vi "Meas Get Record Section.vi"(5 "record index ref":refnum<vi>, 7 "grp index ref":refnum<vi>, 8 "error in":errorcluster, 9 "sub-rec index ref":refnum<vi>, 10 "source mode":T1, 11 "record info":T2={"header path"=path "", "group id"=0, "average id"=0, "Time Stamp"=timestamp(0 s since 1904-01-01), "max samples"=0, "first sample"=0, "first smpl [%]"=-1.0, "kill viewer"=FALSE}) -> (0 "error out":errorcluster, 1 "record path":path, 2 "time [s]":dbl[](array[numeric]), 3 "waveforms [V]":sgl[][](array[numeric]), 4 "labels":string[](array[string]))   [LabVIEW 2020]
doc: "Reads desired section of the record defined in 'record info'. It will read the header file, it will parse it in order to find particular record in it, then it fetches desired portion of the sample data from binary sample file. Then it scales the data using scale factors from the header file."
uses:
  GUI/GUI Waveform Info.ctl
  Meas Sample Reader Source Mode.ctl
  8804b04d-be98-4d58-8b56-90ec7a7b7f07.vi
  octave/infolib/GetI64.vi
  octave/infolib/Get 1D String.vi
  octave/infolib/GetString.vi
  octave/infolib/Get 1D I64.vi
  <vilib>/Comparison/Equal/Equal Functor/Equal Functor.lvclass
  octave/infolib/infolib.lvlib
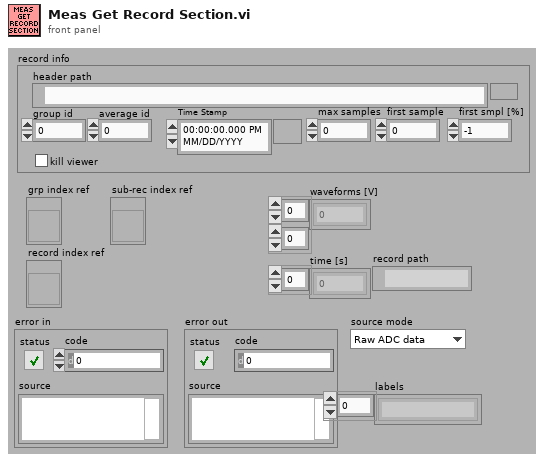
[diagram p1: front panel]
types:
  T1 = typedef "Meas Sample Reader Source Mode.ctl" = enum16{"Raw ADC data", "Transducers"}
  T2 = typedef "GUI Waveform Info.ctl" = cluster{"header path":path, "group id":i32, "average id":i32, "Time Stamp":timestamp, "max samples":i64, "first sample":i64, "first smpl [%]":dbl, "kill viewer":bool}
  T3 = typedef "Corr Transducer INFO Record.ctl" = cluster{"name":string, "serial":string, "channel name":string, "items":T4[], "type":string}
  T4 = typedef "Corr Transducer INFO Item.ctl" = cluster{"name":string, "is numeric":bool, "value":dbl, "uncertainty":dbl, "string value":string, "template":T5, "info":string}
  T5 = typedef "Corr CSV Template.ctl" = cluster{"quantities":string[], "y-axis":string, "x-axis":string}
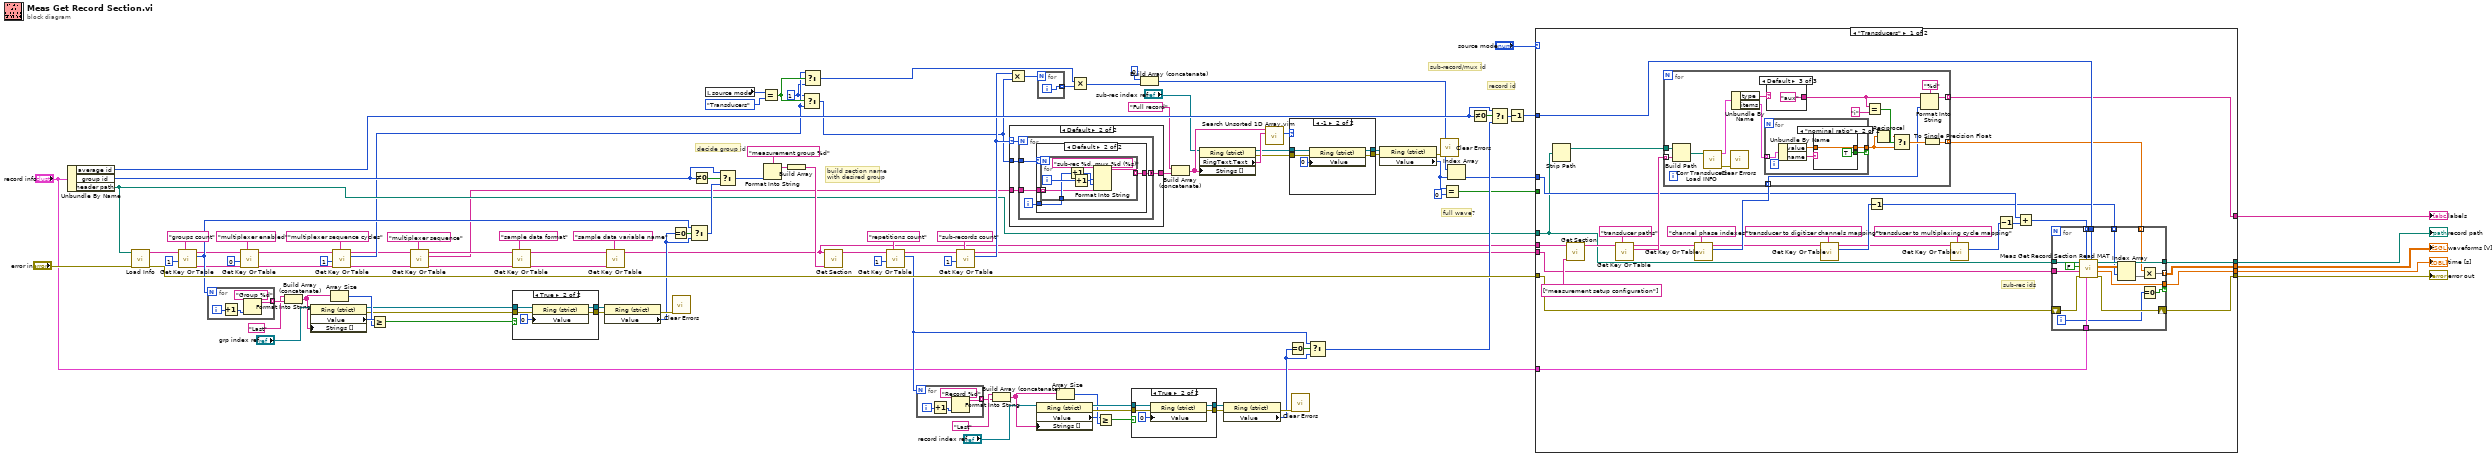
[diagram p0: block diagram]
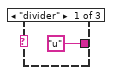
[diagram p3: hidden frame]
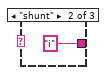
[diagram p4: hidden frame]
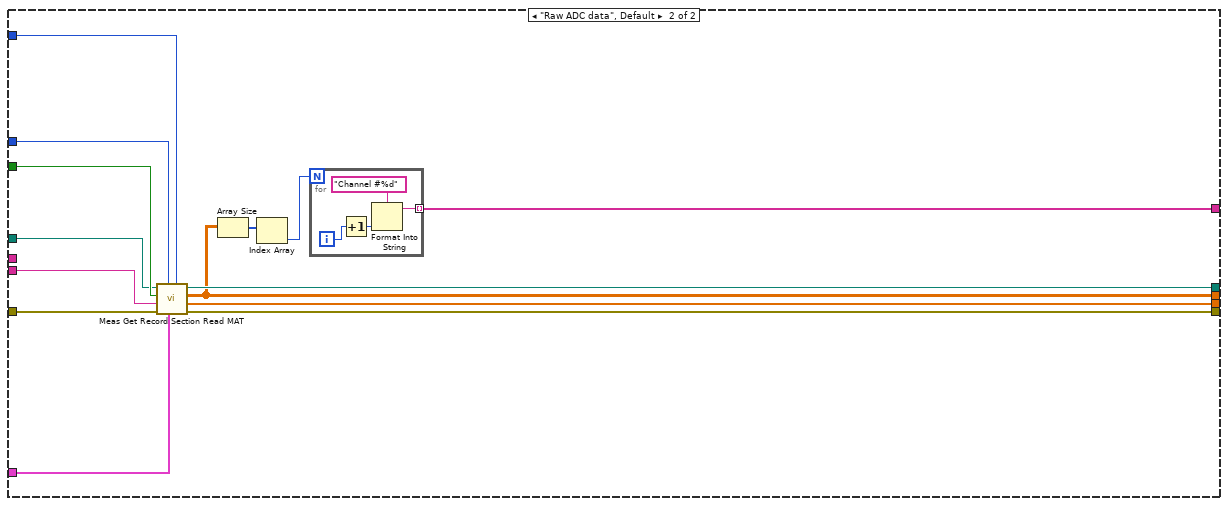
[diagram p5: hidden frame]
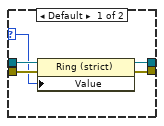
[diagram p6: hidden frame]
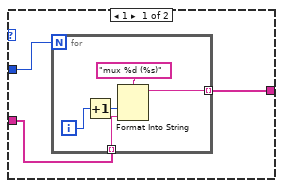
[diagram p7: hidden frame]
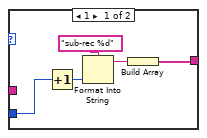
[diagram p8: hidden frame]
diagram:
  w10 = i64 1 ("t")
  # "full wave?"
  # "sub-record/mux id"
  # "record id"
  # "decide group id"
  # "build section name\nwith desired group"
  n1 = Unbundle By Name("record info") -> ("average id"=w97:i32, "group id"=w102:i32, "header path"=w18:path)
  n2 = call "Load Info.vi"("error in"="error in", "filename"=w18) -> ("error out"=w90:errorcluster, "info data"=w106:string)  [unwired: 8 in]
  n3 = call-poly "Get Key Or Table.vi"("key description"="groups count", "numeric"=i64 1, "info data"=w106) -> ("sections out"=w52:string[], "value"=w59:i64, "info data out"=w51:string)  [unwired: 5 in, 1 out]
  n4 = for {
    N: w59 -> [_]
    tunnel: [w111] -> w85 mode=indexing
    i -> [w113]
    n5 = Increment(x=w113) -> (x+1=w110:i32)
    n6 = Format Into String(format string="Group %d", w110) -> (resulting string=w111:string)  [unwired: 2 in, 1 out]
  }
  n7 = call-poly "Get Key Or Table.vi"("key description"="multiplexer enabled", "sections"=w52, "numeric"=i64 0, "info data"=w51) -> ("sections out"=w47:string[], "info data out"=w48:string)  [unwired: 4 in, 2 out]
  n8 = Build Array (concatenate)("Last", w85) -> (w82:string[])
  n9 = property class="Ring (strict)"(reference="grp index ref", "Strings []"=w82) -> (reference out=w80:refnum<vi>, error out=w76:errorcluster, "Value"=w83:u16)  [unwired: 1 in]
  n10 = Array Size(array=w82) -> (size(s)=w81:i32)
  n11 = call-poly "Get Key Or Table.vi"("key description"="multiplexer sequence cycles", "sections"=w47, "numeric"=i64 1, "info data"=w48) -> ("sections out"=w6:string[], "value"=w11:i64, "info data out"=w5:string)  [unwired: 4 in, 1 out]
  n12 = Greater Or Equal?(x=w83, y=w81) -> (x >= y?=w79:bool)
  n13 = call-poly "Get Key Or Table.vi"("key description"="multiplexer sequence", "sections"=w6, "info data"=w5) -> ("sections out"=w3:string[], "value"=w1:string[], "info data out"=w2:string)  [unwired: 5 in, 1 out]
  n14 = call-poly "Get Key Or Table.vi"("key description"="sample data format", "sections"=w3, "info data"=w2) -> ("sections out"=w93:string[], "info data out"=w94:string)  [unwired: 5 in, 2 out]
  n15 = case shown="True" w79 {
    tunnel: w80 -> [w115 w120]
    tunnel: [w115 w118] -> w78
    tunnel: [w114 w117] -> w77
    tunnel: w76 -> [w114 w116]
    frame False {
    }
    frame True {
      n16 = property class="Ring (strict)"(reference=w120, error in=w116, "Value"=u16 0) -> (reference out=w118:refnum<vi>, error out=w117:errorcluster)
    }
  }
  n17 = property class="Ring (strict)"(reference=w78, error in=w77) -> (error out=w75:errorcluster, "Value"=w61:u16)  [unwired: 1 out]
  n18 = call-poly "Get Key Or Table.vi"("key description"="sample data variable name", "sections"=w93, "info data"=w94) -> ("info data out"=w7:string)  [unwired: 5 in, 3 out]
  n19 = Equal To 0?(x=w61) -> (x = 0?=w62:bool)
  n20 = call <vilib>:"Clear Errors.vi"("error in (no error)"=w75) -> ()  [unwired: 5 in, 2 out]
  n21 = Select(t=w59, s=w62, f=w61) -> (s? t:f=w60:i64)
  n22 = Not Equal To 0?(x=w102) -> (x != 0?=w103:bool)
  n23 = local read "source mode"() -> (w14:T1)
  n24 = Select(t=w102, s=w103, f=w60) -> (s? t:f=w101:i64)
  n25 = Equal?(x=w14, y=Meas_Sample_Reader_Source_Mode."Transducers") -> (x = y?=w12:bool)
  n26 = Format Into String(format string="measurement group %d", w101) -> (resulting string=w105:string)  [unwired: 2 in, 1 out]
  n27 = Build Array(w105) -> (w23:string[])
  n28 = Select(t=w10, s=w12, f=w11) -> (s? t:f=w15:i64)
  n29 = Select(t=w11, s=w12, f=w10) -> (s? t:f=w8:i64)
  n30 = call "Get Section.vi"("sections"=w23, "info data"=w7) -> ("section part"=w22:string)  [unwired: 7 in, 2 out]
  n31 = call-poly "Get Key Or Table.vi"("key description"="repetitions count", "numeric"=i64 1, "info data"=w22) -> ("value"=w55:i64, "info data out"=w44:string)  [unwired: 5 in, 2 out]
  n32 = for {
    N: w55 -> [_]
    tunnel: [w122] -> w64 mode=indexing
    i -> [w124]
    n33 = Increment(x=w124) -> (x+1=w121:i32)
    n34 = Format Into String(format string="Record %d", w121) -> (resulting string=w122:string)  [unwired: 2 in, 1 out]
  }
  n35 = call-poly "Get Key Or Table.vi"("key description"="sub-records count", "numeric"=i64 1, "info data"=w44) -> ("value"=w31:i64, "info data out"=w21:string)  [unwired: 5 in, 2 out]
  n36 = Build Array (concatenate)("Last", w64) -> (w67:string[])
  n37 = Multiply(x=w31, y=w15) -> (x*y=w30:i64)
  n38 = case shown="Default" w31 {
    selector: w31 -> [_ w135]
    tunnel: w15 -> [w125 w136]
    tunnel: [w127 w134] -> w43
    tunnel: w1 -> [w126 w133]
    frame 1 {
      n39 = for {
        N: w125 -> [_]
        tunnel: [w130] -> w127 mode=indexing
        tunnel: w126 -> [w128] mode=indexing
        i -> [w129]
        n40 = Increment(x=w129) -> (x+1=w132:i32)
        n41 = Format Into String(format string="mux %d (%s)", w132, w128) -> (resulting string=w130:string)  [unwired: 2 in, 1 out]
      }
    }
    frame Default {
      n42 = for {
        N: w135 -> [_]
        tunnel: w136 -> [w140]
        tunnel: [w138] -> w134 mode=concatenating
        tunnel: w133 -> [w137]
        i -> [w139]
        n43 = case shown="Default" w140 {
          selector: w140 -> [_ w149]
          tunnel: w139 -> [w141 w147]
          tunnel: [w142 w148] -> w138
          tunnel: w137 -> [_ w146]
          frame 1 {
            n44 = Increment(x=w141) -> (x+1=w144:i32)
            n45 = Format Into String(format string="sub-rec %d", w144) -> (resulting string=w143:string)  [unwired: 2 in, 1 out]
            n46 = Build Array(w143) -> (w142:string[])
          }
          frame Default {
            n47 = for {
              N: w149 -> [_]
              tunnel: [w154] -> w148 mode=indexing
              tunnel: w147 -> [w151]
              tunnel: w146 -> [w150] mode=indexing
              i -> [w156]
              n48 = Increment(x=w151) -> (x+1=w152:i32)
              n49 = Increment(x=w156) -> (x+1=w153:i32)
              n50 = Format Into String(format string="sub-rec %d, mux %d (%s)", w152, w153, w150) -> (resulting string=w154:string)  [unwired: 2 in, 1 out]
            }
          }
        }
      }
    }
  }
  n51 = property class="Ring (strict)"(reference="record index ref", "Strings []"=w67) -> (reference out=w69:refnum<vi>, error out=w73:errorcluster, "Value"=w66:u16)  [unwired: 1 in]
  n52 = for {
    N: w30 -> [_]
    tunnel: [w157] -> w29 mode=indexing
    i -> [w157]
  }
  n53 = Array Size(array=w67) -> (size(s)=w68:i32)
  n54 = Multiply(x=w8, y=w29) -> (x*y=w9:i64[])
  n55 = Greater Or Equal?(x=w66, y=w68) -> (x >= y?=w70:bool)
  n56 = case shown="True" w70 {
    tunnel: w69 -> [w159 w164]
    tunnel: [w159 w162] -> w71
    tunnel: [w158 w161] -> w72
    tunnel: w73 -> [w158 w160]
    frame False {
    }
    frame True {
      n57 = property class="Ring (strict)"(reference=w164, error in=w160, "Value"=u16 0) -> (reference out=w162:refnum<vi>, error out=w161:errorcluster)
    }
  }
  n58 = Build Array (concatenate)(0, w9) -> (w28:i64[])
  n59 = Build Array (concatenate)("Full record", w43) -> (w41:string[])
  n60 = property class="Ring (strict)"(reference="sub-rec index ref", "Strings []"=w41) -> (reference out=w36:refnum<vi>, error out=w37:errorcluster, "RingText.Text"=w40:string)  [unwired: 1 in]
  n61 = property class="Ring (strict)"(reference=w71, error in=w72) -> (error out=w74:errorcluster, "Value"=w56:u16)  [unwired: 1 out]
  n62 = call "Search Unsorted 1D Array.vim"("element"=w40, "unsorted 1D array"=w41) -> ("index of element"=w39:i32)  [unwired: 9 in]
  n63 = Equal To 0?(x=w56) -> (x = 0?=w57:bool)
  n64 = case shown="-1" w39 {
    selector: w39 -> [w167 _]
    tunnel: w37 -> [w169 w174]
    tunnel: w36 -> [w168 w173]
    tunnel: [w166 w170] -> w35
    tunnel: [w165 w171] -> w34
    frame Default {
      n65 = property class="Ring (strict)"(reference=w168, error in=w169, "Value"=w167) -> (reference out=w165:refnum<vi>, error out=w166:errorcluster)
    }
    frame -1 {
      n66 = property class="Ring (strict)"(reference=w173, error in=w174, "Value"=u16 0) -> (reference out=w171:refnum<vi>, error out=w170:errorcluster)
    }
  }
  n67 = call <vilib>:"Clear Errors.vi"("error in (no error)"=w74) -> ()  [unwired: 5 in, 2 out]
  n68 = Select(t=w55, s=w57, f=w56) -> (s? t:f=w58:i64)
  n69 = property class="Ring (strict)"(reference=w34, error in=w35) -> (error out=w33:errorcluster, "Value"=w27:u16)  [unwired: 1 out]
  n70 = call <vilib>:"Clear Errors.vi"("error in (no error)"=w33) -> ()  [unwired: 5 in, 2 out]
  n71 = Equal?(x=w27, y=u16 0) -> (x = y?=w19:bool)
  n72 = Index Array(array=w28, index=w27) -> (element=w24:i64)
  n73 = Not Equal To 0?(x=w97) -> (x != 0?=w98:bool)
  n74 = Select(t=w97, s=w98, f=w58) -> (s? t:f=w91:i64)
  n75 = Decrement(x=w91) -> (x-1=w25:i64)
  n76 = case shown="\"Transducers\"" "source mode" {
    tunnel: [w181 w262] -> w92
    tunnel: w90 -> [w187 w261]
    tunnel: [w177 w260] -> w89
    tunnel: [w178 w252] -> w88
    tunnel: [w175 w259] -> w87
    tunnel: w25 -> [w185 w258]
    tunnel: w24 -> [w189 w257]
    tunnel: w21 -> [w183 w256]
    tunnel: "record info" -> [w182 w255]
    tunnel: w19 -> [_ w254]
    tunnel: w18 -> [w184 w253]
    tunnel: [w176 w249] -> w16
    tunnel: w7 -> [w204 _]
    frame "Transducers" {
      # "sub-rec ids"
      n77 = Strip Path(path=w184) -> (stripped path=w201:path)  [unwired: 1 out]
      n78 = call "Get Section.vi"("sections"=string[] ["measurement setup configuration"], "info data"=w204) -> ("section part"=w197:string)  [unwired: 7 in, 2 out]
      n79 = call-poly "Get Key Or Table.vi"("key description"="transducer paths", "info data"=w197) -> ("value"=w200:string[], "info data out"=w198:string)  [unwired: 6 in, 2 out]
      n80 = call-poly "Get Key Or Table.vi"("key description"="channel phase indexes", "info data"=w198) -> ("value"=w196:i64[], "info data out"=w194:string)  [unwired: 6 in, 2 out]
      n81 = for {
        tunnel: w201 -> [w238]
        tunnel: w200 -> [w237] mode=indexing
        tunnel: [w222] -> w179 mode=indexing
        tunnel: w196 -> [w224] mode=indexing
        tunnel: [w223] -> w176 mode=indexing
        n82 = Build Path(base path=w238, name or relative path=w237) -> (appended path=w236:path)
        n83 = call "Corr Transducers Load INFO.vi"("Path"=w236) -> ("error out"=w235:errorcluster, "transducer info"=w234:T3)  [unwired: 9 in]
        n84 = call <vilib>:"Clear Errors.vi"("error in (no error)"=w235) -> ()  [unwired: 5 in, 2 out]
        n85 = Unbundle By Name(w234) -> ("type"=w233:string, "items"=w232:T4[])
        n86 = for {
          tunnel: w232 -> [w243] mode=indexing
          tunnel: [w240] -> w228 if=w239
          n87 = Unbundle By Name(w243) -> ("value"=w241:dbl, "name"=w242:string)
          n88 = case shown="\"nominal ratio\"" w242 {
            tunnel: w241 -> [_ w245]
            tunnel: [_ w245] -> w240
            tunnel: [_ TRUE] -> w239
            frame Default {
            }
            frame "nominal ratio" {
            }
          }
        }
        n89 = case shown="Default" w233 {
          tunnel: ["u" "i" "aux"] -> w226
          frame "divider" {
          }
          frame "shunt" {
          }
          frame Default {
          }
        }
        n90 = Equal?(x=w226, y="i") -> (x = y?=w230:bool)
        n91 = Reciprocal(x=w228) -> (1/x=w229:dbl)
        n92 = Select(t=w229, s=w230, f=w228) -> (s? t:f=w227:dbl)
        n93 = Format Into String(format string="%d", initial string=w226, w224) -> (resulting string=w223:string)  [unwired: 1 in, 1 out]
        n94 = To Single Precision Float(number=w227) -> (single precision float=w222:sgl)
      }
      n95 = call-poly "Get Key Or Table.vi"("key description"="transducer to digitizer channels mapping", "info data"=w194) -> ("value"=w193:i64[], "info data out"=w190:string)  [unwired: 6 in, 2 out]
      n96 = Decrement(x=w193) -> (x-1=w180:i64[])
      n97 = call-poly "Get Key Or Table.vi"("key description"="transducer to multiplexing cycle mapping", "info data"=w190) -> ("value"=w192:i64[])  [unwired: 6 in, 3 out]
      n98 = Decrement(x=w192) -> (x-1=w188:i64[])
      n99 = Add(x=w189, y=w188) -> (x+y=w186:i64[])
      n100 = for {
        tunnel: w186 -> [w220] mode=indexing
        tunnel: w185 -> [w219]
        tunnel: w183 -> [w216]
        tunnel: w182 -> [w215]
        tunnel: w180 -> [w212] mode=indexing
        tunnel: w179 -> [w210] mode=indexing
        tunnel: [w209] -> w178 mode=indexing
        tunnel: [w208] -> w175 if=w206
        shift-right: [w207] -> w177
        shift-left: w187 -> [w221]
        tunnel: w184 -> [w218]
        tunnel: [w214] -> w181
        i -> [w205]
        n101 = call "Meas Get Record Section Read MAT.vi"("record id"=w219, "record position info"=w215, "sub-record id"=w220, "error in (no error)"=w221, "info data in"=w216, "full wave or sub-record? (T: full wave)"=FALSE, "meas header path"=w218) -> ("error out"=w207:errorcluster, "time vector [s]"=w208:dbl[], "waveform(s)"=w213:sgl[][], "raw MAT path"=w214:path)  [unwired: 1 in]
        n102 = Index Array(array=w213, index (row)=w212) -> (element=w211:sgl[])  [unwired: 1 in]
        n103 = Multiply(x=w210, y=w211) -> (x*y=w209:sgl[])
        n104 = Equal To 0?(x=w205) -> (x = 0?=w206:bool)
      }
    }
    frame "Raw ADC data", Default {
      n105 = call "Meas Get Record Section Read MAT.vi"("record id"=w258, "record position info"=w255, "sub-record id"=w257, "error in (no error)"=w261, "info data in"=w256, "full wave or sub-record? (T: full wave)"=w254, "meas header path"=w253) -> ("error out"=w260:errorcluster, "time vector [s]"=w259:dbl[], "waveform(s)"=w252:sgl[][], "raw MAT path"=w262:path)  [unwired: 1 in]
      n106 = Array Size(array=w252) -> (size(s)=w251:i32[])
      n107 = Index Array(array=w251) -> (element=w250:i32)  [unwired: 1 in]
      n108 = for {
        N: w250 -> [_]
        tunnel: [w263] -> w249 mode=indexing
        i -> [w264]
        n109 = Increment(x=w264) -> (x+1=w265:i32)
        n110 = Format Into String(format string="Channel #%d", w265) -> (resulting string=w263:string)  [unwired: 2 in, 1 out]
      }
    }
  }
  "error out" <- w89
  "waveforms [V]" <- w88
  "time [s]" <- w87
  "record path" <- w92
  "labels" <- w16
